vi "Replace_(X,Y,dX,dY)_to_Specified_Number-2.vi"(2 "Starting index":i32, 3 "Replacement \nnumber":dbl, 4 "[IN] Sample \narray":dbl[](array[numeric])) -> (0 "Finishing index":i32, 1 "[OUT] Processed\narray":dbl[](array[numeric]))   [LabVIEW 2017]
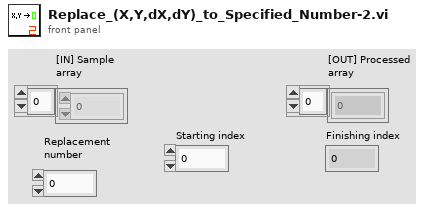
[diagram p1: front panel]
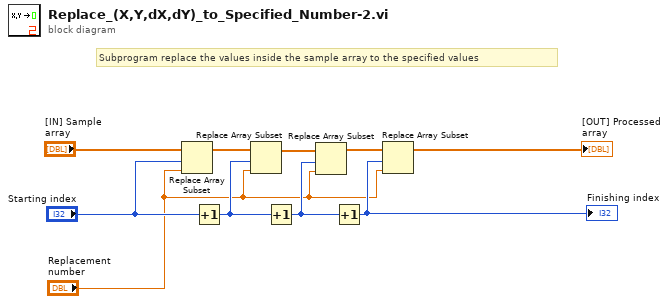
[diagram p0: block diagram]
diagram:
  # "Subprogram replace the values inside the sample array to the specified values"
  n1 = Replace Array Subset(array="[IN] Sample \narray", new element="Replacement \nnumber", index="Starting index") -> (w9:dbl[])
  n2 = Increment(x="Starting index") -> (x+1=w6:i32)
  n3 = Replace Array Subset(array=w9, new element="Replacement \nnumber", index=w6) -> (w7:dbl[])
  n4 = Increment(x=w6) -> (x+1=w4:i32)
  n5 = Replace Array Subset(array=w7, new element="Replacement \nnumber", index=w4) -> (w5:dbl[])
  n6 = Increment(x=w4) -> (x+1=w3:i32)
  "Finishing index" <- w3
  n7 = Replace Array Subset(array=w5, new element="Replacement \nnumber", index=w3) -> (→"[OUT] Processed\narray":dbl[])
